vi "cRIO-HMI Communication.vi"(8 "error in (no error)":errorcluster, 11 "Message Queue":refnum<queue>) -> (0 "error out":errorcluster)   [LabVIEW 2021]
uses:
  Controls/RT Network States.ctl
  support/Message Queue/Message Cluster.ctl
  Global Variables/Network Globals.vi
  Global Variables/RT GV.vi
  support/Message Queue/Enqueue Message (Single).vi
  support/Message Queue/Message Queue.lvlib
panel:
  in  "MissedHB":i32=3
  out "State":T1
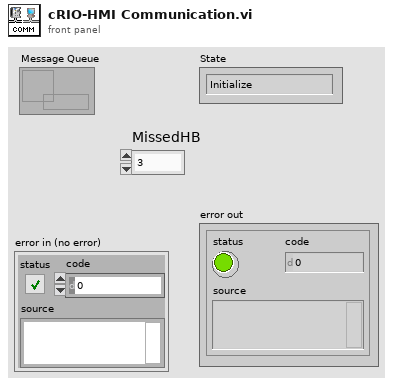
[diagram p1: front panel]
types:
  T1 = typedef "RT Network States.ctl" = enum16{"Initialize", "Connect", "Connected"}
  T2 = cluster{"Message":string, "Message Data":variant}
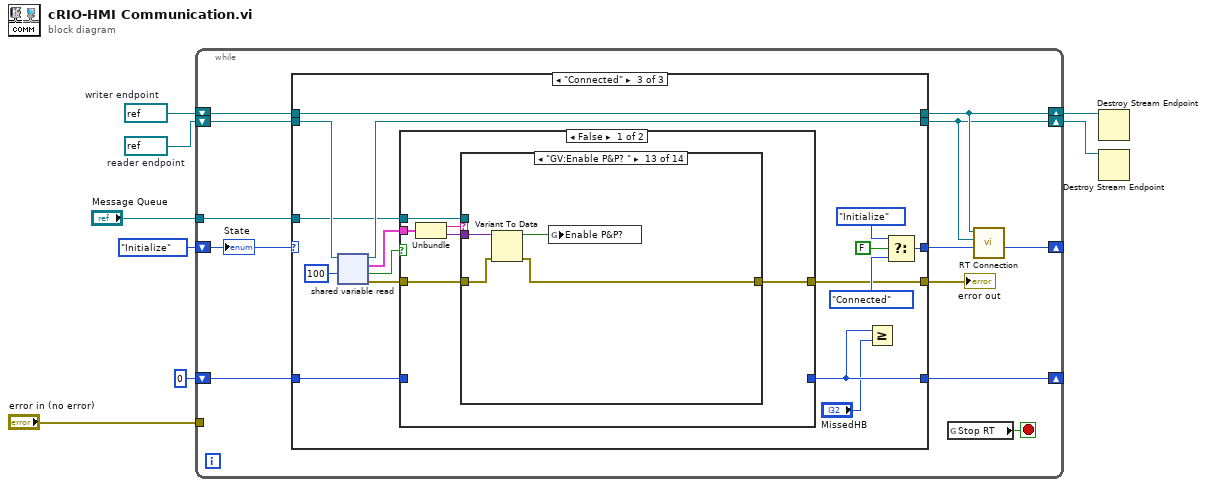
[diagram p0: block diagram]
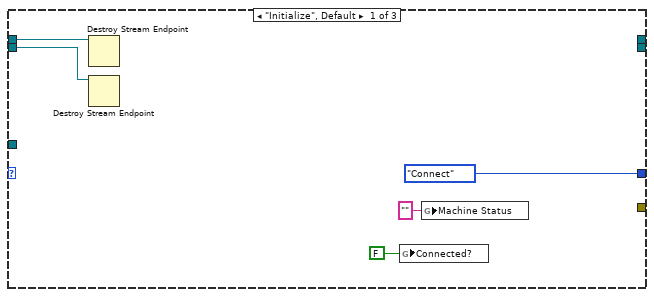
[diagram p2: hidden frame]
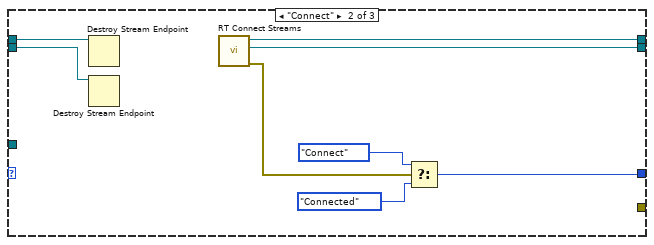
[diagram p3: hidden frame]
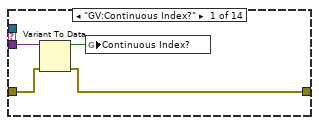
[diagram p4: hidden frame]
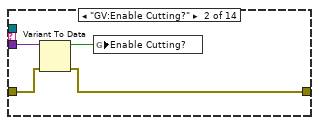
[diagram p5: hidden frame]
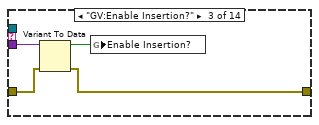
[diagram p6: hidden frame]
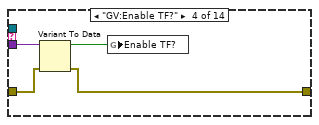
[diagram p7: hidden frame]
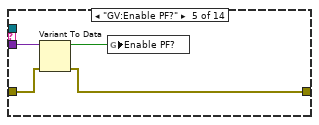
[diagram p8: hidden frame]
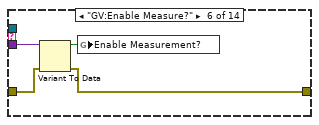
[diagram p9: hidden frame]
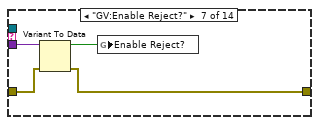
[diagram p10: hidden frame]
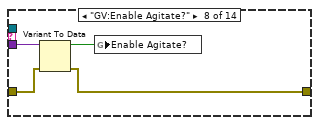
[diagram p11: hidden frame]
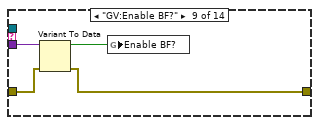
[diagram p12: hidden frame]
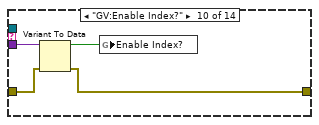
[diagram p13: hidden frame]
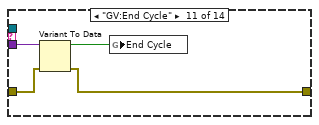
[diagram p14: hidden frame]
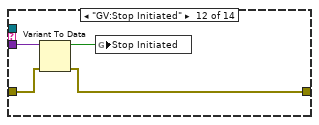
[diagram p15: hidden frame]
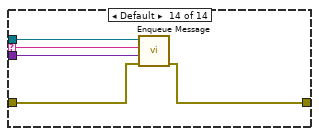
[diagram p16: hidden frame]
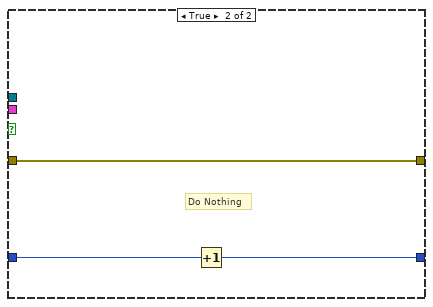
[diagram p17: hidden frame]
diagram:
  w7 = refnum<k21> refnum  # reader endpoint
  w6 = refnum<k21> refnum  # writer endpoint
  n1 = while {
    shift-right: [w15] -> w4
    shift-left: w6 -> [w19]
    shift-right: [w14] -> w5
    shift-left: w7 -> [w18]
    shift-right: [w16] -> _
    shift-left: RT_Network_States."Initialize" -> [w20]
    tunnel: "error in (no error)" -> [_]
    shift-right: [w11] -> _
    shift-left: 0 -> [w12]
    tunnel: "Message Queue" -> [w9]
    stop <- w10 stop-if-true
    n2 = case shown="\"Connected\"" w20 {
      tunnel: [_ w32 w49] -> w15
      tunnel: [_ w31 w46] -> w14
      tunnel: w19 -> [w25 w27 w49]
      tunnel: w18 -> [w24 w26 w47]
      tunnel: [RT_Network_States."Connect" w33 w40] -> w17
      tunnel: [_ _ w35] -> w13
      tunnel: w12 -> [_ _ w43]
      tunnel: [_ _ w42] -> w11
      tunnel: w9 -> [_ _ w34]
      frame "Initialize", Default {
        n3 = Destroy Stream Endpoint(11:w25) -> ()  [unwired: 1 in, 1 out]
        n4 = Destroy Stream Endpoint(11:w24) -> ()  [unwired: 1 in, 1 out]
        n5 = global write "Network Globals.vi" "Connected?"(FALSE ("Stop RT")) -> ()
        n6 = global write "RT GV.vi" "Machine Status"("" ("Machine Status")) -> ()
      }
      frame "Connect" {
        n7 = Destroy Stream Endpoint(11:w27) -> ()  [unwired: 1 in, 1 out]
        n8 = Destroy Stream Endpoint(11:w26) -> ()  [unwired: 1 in, 1 out]
        n9 = call "RT Connect Streams.vi"() -> ("error out"=w28:errorcluster, "reader endpoint"=w31:refnum<k21>, "writer endpoint"=w32:refnum<k21>)  [unwired: 9 in]
        n10 = Select(t=RT_Network_States."Connect", s=w28, f=RT_Network_States."Connected") -> (s? t:f=w33:T1)
      }
      frame "Connected" {
        n11 = shared-variable-read(w47, 100 ("timeout ms (-1)")) -> (w46:refnum<k21>, w36:errorcluster, w45:bool, w44:T2)  [unwired: 1 in]
        n12 = case shown="False" w45 {
          tunnel: w44 -> [w55 _]
          tunnel: w43 -> [_ w115]
          tunnel: [_ w114] -> w42
          tunnel: w36 -> [w52 w113]
          tunnel: [w51 w113] -> w35
          tunnel: w34 -> [w50 _]
          frame False {
            n13 = Unbundle(w55) -> ("Message"=w54:string, "Message Data"=w53:variant)
            n14 = case shown="\"GV:Enable P&P? \"" w54 {
              selector: w54 -> [_ _ _ _ _ _ _ _ _ _ _ _ _ w112]
              tunnel: w53 -> [w59 w63 w67 w71 w75 w79 w83 w87 w91 w95 w99 w103 w107 w111]
              tunnel: w52 -> [w58 w62 w66 w70 w74 w78 w82 w86 w90 w94 w98 w102 w106 w110]
              tunnel: [w57 w61 w65 w69 w73 w77 w81 w85 w89 w93 w97 w101 w105 w109] -> w51
              tunnel: w50 -> [_ _ _ _ _ _ _ _ _ _ _ _ _ w108]
              frame "GV:Continuous Index?" {
                n15 = Variant To Data(error in=w58, Variant=w59) -> (data=w56:bool, error out=w57:errorcluster)  [unwired: 1 in]
                n16 = global write "RT GV.vi" "Continuous Index?"(w56) -> ()
              }
              frame "GV:Enable Cutting?" {
                n17 = Variant To Data(error in=w62, Variant=w63) -> (data=w60:bool, error out=w61:errorcluster)  [unwired: 1 in]
                n18 = global write "RT GV.vi" "Enable Cutting?"(w60) -> ()
              }
              frame "GV:Enable Insertion?" {
                n19 = Variant To Data(error in=w66, Variant=w67) -> (data=w64:bool, error out=w65:errorcluster)  [unwired: 1 in]
                n20 = global write "RT GV.vi" "Enable Insertion?"(w64) -> ()
              }
              frame "GV:Enable TF?" {
                n21 = Variant To Data(error in=w70, Variant=w71) -> (data=w68:bool, error out=w69:errorcluster)  [unwired: 1 in]
                n22 = global write "RT GV.vi" "Enable TF?"(w68) -> ()
              }
              frame "GV:Enable PF?" {
                n23 = Variant To Data(error in=w74, Variant=w75) -> (data=w72:bool, error out=w73:errorcluster)  [unwired: 1 in]
                n24 = global write "RT GV.vi" "Enable PF?"(w72) -> ()
              }
              frame "GV:Enable Measure?" {
                n25 = Variant To Data(error in=w78, Variant=w79) -> (data=w76:bool, error out=w77:errorcluster)  [unwired: 1 in]
                n26 = global write "RT GV.vi" "Enable Measurement?"(w76) -> ()
              }
              frame "GV:Enable Reject?" {
                n27 = Variant To Data(error in=w82, Variant=w83) -> (data=w80:bool, error out=w81:errorcluster)  [unwired: 1 in]
                n28 = global write "RT GV.vi" "Enable Reject?"(w80) -> ()
              }
              frame "GV:Enable Agitate?" {
                n29 = Variant To Data(error in=w86, Variant=w87) -> (data=w84:bool, error out=w85:errorcluster)  [unwired: 1 in]
                n30 = global write "RT GV.vi" "Enable Agitate?"(w84) -> ()
              }
              frame "GV:Enable BF?" {
                n31 = Variant To Data(error in=w90, Variant=w91) -> (data=w88:bool, error out=w89:errorcluster)  [unwired: 1 in]
                n32 = global write "RT GV.vi" "Enable BF?"(w88) -> ()
              }
              frame "GV:Enable Index?" {
                n33 = Variant To Data(error in=w94, Variant=w95) -> (data=w92:bool, error out=w93:errorcluster)  [unwired: 1 in]
                n34 = global write "RT GV.vi" "Enable Index?"(w92) -> ()
              }
              frame "GV:End Cycle" {
                n35 = Variant To Data(error in=w98, Variant=w99) -> (data=w96:bool, error out=w97:errorcluster)  [unwired: 1 in]
                n36 = global write "RT GV.vi" "End Cycle"(w96) -> ()
              }
              frame "GV:Stop Initiated" {
                n37 = Variant To Data(error in=w102, Variant=w103) -> (data=w100:bool, error out=w101:errorcluster)  [unwired: 1 in]
                n38 = global write "RT GV.vi" "Stop Initiated"(w100) -> ()
              }
              frame "GV:Enable P&P? " {
                n39 = Variant To Data(error in=w106, Variant=w107) -> (data=w104:bool, error out=w105:errorcluster)  [unwired: 1 in]
                n40 = global write "RT GV.vi" "Enable P&P?"(w104) -> ()
              }
              frame Default {
                n41 = call-poly "Enqueue Message.vi"("error in (no error)"=w110, "Message Data"=w111, "Message"=w112, "Message Queue"=w108) -> ("error out"=w109:errorcluster)  [unwired: 6 in, 1 out]
              }
            }
          }
          frame True {
            # "Do Nothing"
            n42 = Increment(x=w115) -> (x+1=w114:i32)
          }
        }
        n43 = Greater Or Equal?(x=w42, y="MissedHB") -> ()  [unwired: 1 out]
        n44 = Select(t=RT_Network_States."Initialize", s=FALSE, f=RT_Network_States."Connected") -> (s? t:f=w40:T1)
      }
    }
    "error out" <- w13
    n45 = global read "Network Globals.vi" "Stop RT"() -> (w10:bool)
    n46 = call "RT Connection.vi"("Next State in"=w17, "reader endpoint"=w14, "writer endpoint"=w15) -> ("Next State out"=w16:T1)  [unwired: 8 in]
    "State" <- w20
  }
  n47 = Destroy Stream Endpoint(11:w4) -> ()  [unwired: 1 in, 1 out]
  n48 = Destroy Stream Endpoint(11:w5) -> ()  [unwired: 1 in, 1 out]
